vi "XML_Decode XML encoded string.vi"(4 "String in":string) -> (1 "String out":string)   [LabVIEW 2011, in "XML Parser.lvlib"]
doc: "This VI replaces XML-encoded (ampersand-encoded) characters with their unencoded counterparts.\n\nThe following character combinations are converted:\n\n&quot; -> \"\n&lt; -> <\n&gt; -> >\n&apos; -> '\n&amp; -> &"
uses:
  XML Parser.lvlib
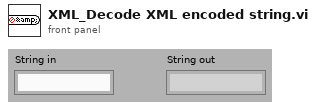
[diagram p1: front panel]
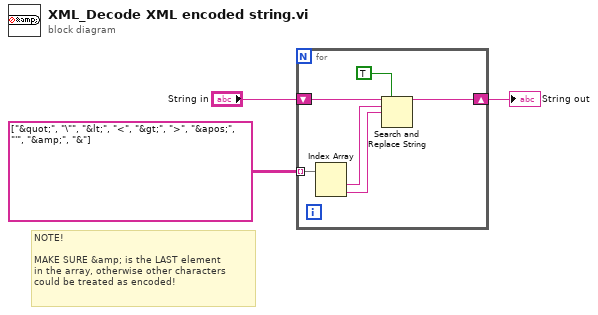
[diagram p0: block diagram]
diagram:
  # "NOTE!\n\nMAKE SURE &amp; is the LAST element\nin the array, otherwise other characters\ncould be treated as encoded!"
  n1 = for {
    tunnel: string[][] [["&quot;", "\""], ["&lt;", "<"], ["&gt;", ">"], ["&apos;", "'"], ["&amp;", "&"]] -> [w9] mode=indexing
    shift-right: [w4] -> w1
    shift-left: "String in" -> [w8]
    n2 = Index Array(array=w9) -> (element #1=w7:string, element #2=w6:string)  [unwired: 2 in]
    n3 = Search and Replace String(replace all?=TRUE ("replace all? (F)"), input string=w8, search string=w7, replace string=w6) -> (result string=w4:string)  [unwired: 4 in, 3 out]
  }
  "String out" <- w1
